vi "subDFD_Find IWL for Coef.vi"(11 "coefficients":dbl[](array[numeric])) -> (3 "iwl":i16)   [LabVIEW 2017]
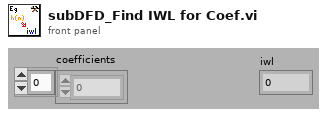
[diagram p1: front panel]
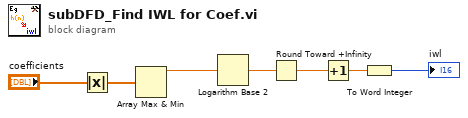
[diagram p0: block diagram]
diagram:
  n1 = Absolute Value(x="coefficients") -> (abs(x)=w6:dbl[])
  n2 = Array Max & Min(array=w6) -> (max value=w5:dbl)  [unwired: 3 out]
  n3 = Logarithm Base 2(1:w5) -> (0:w4:dbl)
  n4 = Round Toward +Infinity(x=w4) -> (ceil(x): smallest int >= x=w3:dbl)
  n5 = Increment(x=w3) -> (x+1=w2:dbl)
  n6 = To Word Integer(number=w2) -> (16bit integer=→"iwl":i16)
